vi "PH_Sixpack.Move.vi"(0 "i ref in":refnum<vi>, 1 "axis":i32=-1, 4 "Device Error in":errorcluster, 5 "error in":errorcluster) -> (14 "i ref out":refnum<vi>, 18 "Device Error out":errorcluster, 19 "error out":errorcluster)   [LabVIEW 2014, in "PH_Sixpack.lvlib"]
doc: "This VI starts ramping or a reference search."
uses:
  PH_Sixpack.lvlib
  instr.lib/Sixpack/Sixpack - Driver.lvlib
  PH_Basics/PH_Stepmotor_BaseClass/PH_Stepmotor_BaseClass.lvlib
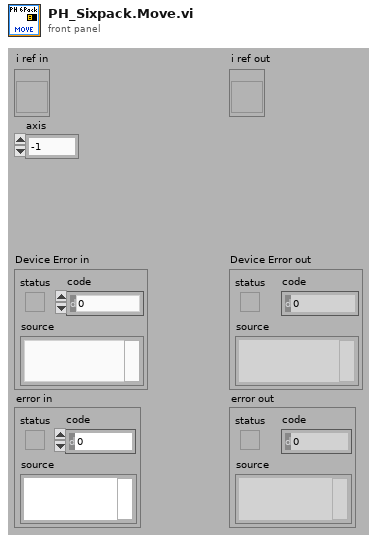
[diagram p1: front panel]
types:
  T1 = typedef "PH_Stepmotor_BaseClass.lvlib/PH_Stepmotor_BaseClass.Axis Attributes.ctl" = cluster{"Settings":T2, "Endswitch?":bool, "DIM Service IDs":T4, "Activity":T5, "Configured?":bool, "Position":cluster{"Current":i32, "Target":i32}, "Position to set":cluster{"New?":bool, "Wanted":i32}, "Stop?":bool, "Reset?":bool, "Move?":bool, "Nothing connected?":bool}
  T2 = typedef "PH_Stepmotor_BaseClass.lvlib/PH_Stepmotor_BaseClass.Axis Settings.ctl" = cluster{"Sign change":bool, "Width":dbl, "Calibration":dbl, "Unit":string, "Motor Type":T3, "Unit Width":string, "Unit CF":string}
  T3 = typedef "PH_Stepmotor_BaseClass.lvlib/PH_Stepmotor_BaseClass.Motor Type.ctl" = enum16{"Unspecific", "OWIS 49.120.2633", "OWIS 49.060.1033", "OWIS 43.040.2558", "Diamond Motion 2200 series", "OWIS 49.120.266B.MV6", "Calorimeter", "Linear Stage 1", "MICOS VT-80", "MICOS VT-80 S", "Standa Rotstage nt0.95A", "PUF RA 320.200", "PUF RA 800.200", "PUF RA 800.400", "PUF RA 400.50", "1324.nn.800.50", "1324.n9c.800.50", "1324.nn.320.200", "1324.nn.400.200", "1324.nn.800.200", "1324.nn.400.50", "1324.8c9c.800.50", "1324.8c9c.400.200"}
  T4 = typedef "PH_Stepmotor_BaseClass.lvlib/PH_Stepmotor_BaseClass.Axis DIM Service IDs.ctl" = cluster{"Settings":i32, "Information":i32}
  T5 = typedef "PH_Stepmotor_BaseClass.lvlib/PH_Stepmotor_BaseClass.Axis Activity.ctl" = enum16{"No Information", "stopped", "running", "Failure", "Alarm", "stopped at backward ES", "stopped at foreward ES"}
  T6 = typedef "PH_Sixpack.lvlib/PH_Sixpack.Axis Cluster.ctl" = cluster{"Config":T7, "To set?":cluster{"VmaxAmax":bool, "I max":bool, "VStartVminDivi":bool, "Ref Search Parameter":bool, "Stopswitch Limits":bool, "Axis Parameter":bool, "I Control":bool}}
  T7 = typedef "PH_Sixpack.lvlib/PH_Sixpack.Axis Configuration.ctl" = cluster{"VmaxAmax":T8, "I max (50%)":T9, "VStartVminDivi":T10, "Ref Search Parameter":T11, "Stopswitch Limits":T12, "Axis Parameter":T13, "I Control":T16}
  T8 = typedef "Sixpack - Driver.lvlib/VmaxAmax.ctl" = cluster{"VMax(511)":u16, "AMax(128)":u16}
  T9 = typedef "Sixpack - Driver.lvlib/PeakCurrent.ctl" = dbl
  T10 = typedef "Sixpack - Driver.lvlib/VStartVmin.ctl" = cluster{"VStart(5)":u16, "Vmin(4)":u16, "Div i (2)":enum8{"0", "1", "2", "3"}}
  T11 = typedef "Sixpack - Driver.lvlib/Ref Search Parameter.ctl" = cluster{"VRefMax(100)":u16, "DebouncingTime (22ms)":u8}
  T12 = typedef "Sixpack - Driver.lvlib/Stopswitch Limits.ctl" = cluster{"MinLeft(0)":u16, "MaxRight(1023)":u16}
  T13 = typedef "Sixpack - Driver.lvlib/Motor Parameter.ctl" = cluster{"Poslimit (6400)":u32, "P5 Bits":T14, "P6 Bits":T15}
  T14 = typedef "Sixpack - Driver.lvlib/MotorParameter_P5.ctl" = cluster{"MT_PI":bool, "MT_ROTARY":bool, "MT_AUTONULLCMD":bool, "MT_TESTNULL":bool, "MT_NULLLEFT":bool, "MT_NULLCENTRE":bool, "MT_STOPNULL":bool, "MT_FILTERSWITCH":bool}
  T15 = typedef "Sixpack - Driver.lvlib/MotorParameter_P6.ctl" = cluster{"MT_OPTIMIZEWAY":bool, "MT_FASTREF":bool, "MT_MECHREF":bool, "MT_DELAYTESTNULL":bool, "MT_STOPSOFT":bool, "MT_STOPNOREF":bool, "MT_NULLPOSITIVE":bool, "MUT_STOPFULSTEPS":bool}
  T16 = typedef "Sixpack - Driver.lvlib/Current Control.ctl" = cluster{"PowerDownDelay (500)":u16, "PowerDown (0%)":T17, "Standing (50%)":T17, "Running (75%)":T17, "Accelerating (100%)":T17}
  T17 = typedef "Sixpack - Driver.lvlib/Current.ctl" = enum8{"100%", "75%", "50%", "38%", "25%", "19%", "13%", "9%", "0%"}
  T18 = cluster{"VmaxAmax":bool, "I max":bool, "VStartVminDivi":bool, "Ref Search Parameter":bool, "Stopswitch Limits":bool, "Axis Parameter":bool, "I Control":bool}
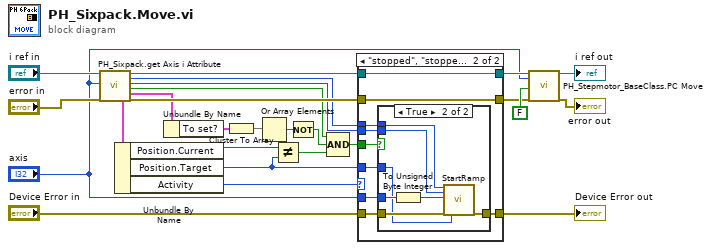
[diagram p0: block diagram]
diagram:
  n1 = call "PH_Sixpack.get Axis i Attribute.vi"("VI in"="i ref in", "Axis"="axis", "error in"="error in") -> ("Axis Base Class Attributes"=w15:T1, "VI out"=w22:refnum<vi>, "HANDLE"=w20:i32, "SixPack ID(0)"=w19:u16, "Axis found?"=w9:bool, "Axis Attributes"=w14:T6, "error out"=w21:errorcluster)  [unwired: 10 in]
  n2 = Unbundle By Name(w15) -> ("Position.Current"=w12:i32, "Position.Target"=w7:i32, "Activity"=w13:T5)
  n3 = Unbundle By Name(w14) -> ("To set?"=w18:T18)
  n4 = Cluster To Array(cluster=w18) -> (array=w17:bool[])
  n5 = Or Array Elements(Boolean array=w17) -> (logical OR=w16:bool)
  n6 = Not Equal?(x=w12, y=w7) -> (x != y?=w8:bool)
  n7 = Not(x=w16) -> (.not. x?=w11:bool)
  n8 = Compound Arithmetic op=AND(w9, w11, w8) -> (w6:bool)
  n9 = case shown="\"stopped\", \"stopped at backward ES\", \"stopped at foreward ES\"" w13 {
    tunnel: [w29 w33] -> w4
    tunnel: [w28 w32] -> w2
    tunnel: [w27 w38] -> w24
    tunnel: "Device Error in" -> [w27 w37]
    tunnel: w22 -> [w29 w33]
    tunnel: w21 -> [w28 w32]
    tunnel: w20 -> [_ w36]
    tunnel: w19 -> [_ w35]
    tunnel: "axis" -> [_ w34]
    tunnel: w7 -> [_ w31]
    tunnel: w6 -> [_ w30]
    frame "No Information", Default {
    }
    frame "stopped", "stopped at backward ES", "stopped at foreward ES" {
      n10 = case shown="True" w30 {
        tunnel: [w39 w46] -> w38
        tunnel: w37 -> [w39 w45]
        tunnel: w36 -> [_ w43]
        tunnel: w35 -> [_ w42]
        tunnel: w34 -> [_ w41]
        tunnel: w31 -> [_ w40]
        frame False {
        }
        frame True {
          n11 = To Unsigned Byte Integer(number=w41) -> (unsigned 8bit integer=w44:u8)
          n12 = call "StartRamp.vi"("handle in"=w43, "UnitAddress(0)"=w42, "MotNr(0)"=w44, "error in"=w45, "TargetPosition(0)"=w40) -> ("error out"=w46:errorcluster)  [unwired: 13 in, 1 out]
        }
      }
    }
  }
  "Device Error out" <- w24
  n13 = call "PH_Stepmotor_BaseClass.PC Move.vi"("i ref in"=w4, "axis"="axis", "Move"=FALSE, "error in (no error)"=w2) -> ("i ref out"=→"i ref out":refnum<vi>, "error out"=→"error out":errorcluster)  [unwired: 14 in]
